vi "ConfigLCR.vi"(0 "Input parameters":T1={"Measurement type"=enum."Test", "Sensor type"=enum."HPK_8in_256", "Identifier"="test.txt", "Open after execution?"=FALSE, "Plot after execution?"=FALSE, "Display channel"=0, "Voltage Delay (s)"=0.5, "Switch Delay (s)"=0.01, "VISA resource name source"="", "VISA resource name DMM"="", "VISA resource name LCR"="", "Compliance  Level (uA)"=10.0, "Voltage Limit (V)"=1000.0, "Data storage location"="", "Scan voltages"="", "Use source as DMM?"=FALSE, "Single channel?"=FALSE, "LCR signal frequenzy (Hz)"=10.0, "DMM device"=enum."Keithley2001", "Sampling number"=1, "Use env. sensors on"=enum."Sensirion sht1x/7x"} {"Voltage Limit (V)" format="%#_13g"; "Voltage Delay (s)" format="%#_13g"; "Switch Delay (s)" format="%#_13g"}, 11 "error in (no error)":errorcluster) -> (4 "VISA resource name out":refnum<visa-resource-name>, 15 "error out":errorcluster)   [LabVIEW 2016]
uses:
  Input_parameters.ctl
  instr.lib/Agilent E4980/Agilent E4980.lvlib
panel:
  in  "Signal Frequency (1000 Hz)":dbl=10000.0
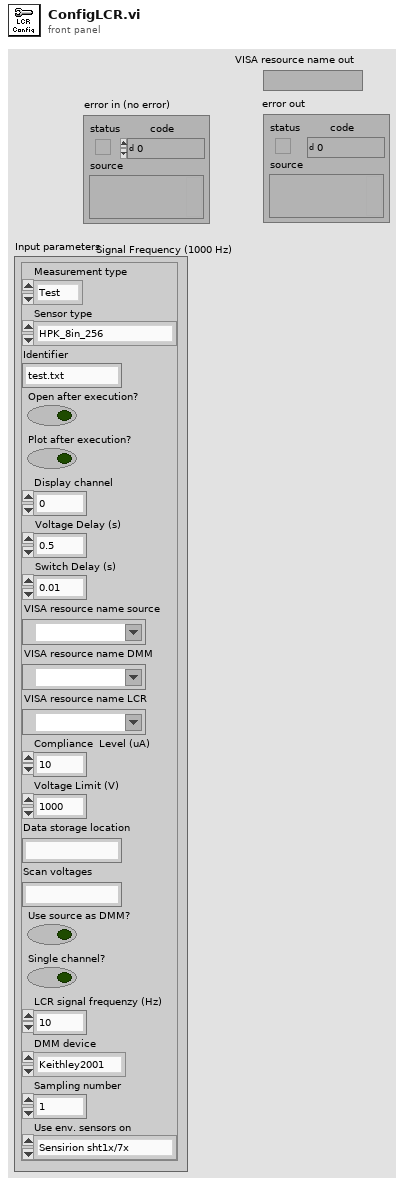
[diagram p1: front panel]
types:
  T1 = typedef "Input_parameters.ctl" = cluster{"Measurement type":enum16{"IV", "CV", "Test"}, "Sensor type":enum16{"HPK_6in_135", "HPK_8in_256", "INF_8in_256", "Diode", "HPK_6in_256"}, "Identifier":string, "Open after execution?":bool, "Plot after execution?":bool, "Display channel":i32, "Voltage Delay (s)":dbl, "Switch Delay (s)":dbl, "VISA resource name source":refnum<visa-resource-name>, "VISA resource name DMM":refnum<visa-resource-name>, "VISA resource name LCR":refnum<visa-resource-name>, "Compliance  Level (uA)":dbl, "Voltage Limit (V)":dbl, "Data storage location":string, "Scan voltages":string, "Use source as DMM?":bool, "Single channel?":bool, "LCR signal frequenzy (Hz)":dbl, "DMM device":enum16{"Keithley2001", "Keithley2450", "Keithley2410"}, "Sampling number":i32, "Use env. sensors on":enum16{"Sensirion sht1x/7x", "Switch Matrix", "Probecard"}}
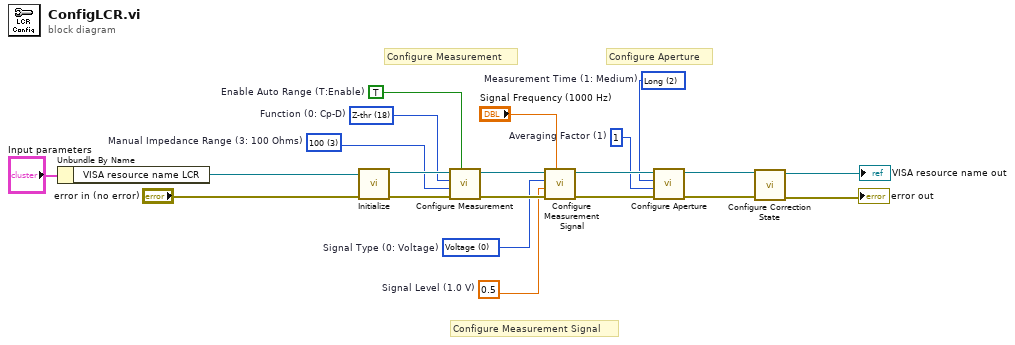
[diagram p0: block diagram]
diagram:
  w10 = u16 2 items=["Short", "Medium", "Long"]  # Measurement Time (1: Medium)
  w9 = 1  # Averaging Factor (1)
  w11 = 0.5  # Signal Level (1.0 V)
  w12 = u16 0 items=["Voltage", "Current"]  # Signal Type (0: Voltage)
  w13 = 3 items=["100m", "1", "10", "100", "300", "1K", "3K", "10K", "30K", "100K"]  # Manual Impedance Range (3: 100 Ohms)
  w14 = u16 18 items=["Cp-D", "Cp-Q", "Cp-G", "Cp-Rp", "Cs-D", "Cs-Q", "Cs-Rs", "Lp-D", "Lp-Q", "Lp-G", "Lp-Rp", "Lp-Rdc", "Ls-D", "Ls-Q", "Ls-Rs", "Ls-Rdc", "R-X", "Z-thd", "Z-thr", "G-B", "Y-thd", "Y-thr", "Vdc-Idc"]  # Function (0: Cp-D)
  w15 = TRUE  # Enable Auto Range (T:Enable)
  # "Configure Aperture"
  # "Configure Measurement Signal"
  # "Configure Measurement"
  n1 = Unbundle By Name("Input parameters") -> ("VISA resource name LCR"=w1:refnum<visa-resource-name>)
  n2 = call "Initialize.vi"("error in (no error)"="error in (no error)", "VISA resource name"=w1) -> ("error out"=w20:errorcluster, "VISA resource name out"=w21:refnum<visa-resource-name>)  [unwired: 8 in]
  n3 = call "Configure Measurement.vi"("Enable Auto Range (T:Enable)"=w15, "error in (no error)"=w20, "Manual Impedance Range (3: 100 Ohms)"=w13, "Function (0: Cp-D)"=w14, "VISA resource name"=w21) -> ("error out"=w18:errorcluster, "VISA resource name out"=w19:refnum<visa-resource-name>)  [unwired: 5 in]
  n4 = call "Configure Measurement Signal.vi"("Signal Frequency (1000 Hz)"="Signal Frequency (1000 Hz)", "error in (no error)"=w18, "Signal Level (1.0 V)"=w11, "Signal Type (0: Voltage)"=w12, "VISA resource name"=w19) -> ("error out"=w16:errorcluster, "VISA resource name out"=w17:refnum<visa-resource-name>)  [unwired: 5 in]
  n5 = call "Configure Aperture.vi"("error in (no error)"=w16, "Averaging Factor (1)"=w9, "Measurement Time (1: Medium)"=w10, "VISA resource name"=w17) -> ("error out"=w7:errorcluster, "VISA resource name out"=w5:refnum<visa-resource-name>)  [unwired: 6 in]
  n6 = call "Configure Correction State.vi"("error in (no error)"=w7, "VISA resource name"=w5) -> ("error out"=→"error out":errorcluster, "VISA resource name out"=→"VISA resource name out":refnum<visa-resource-name>)  [unwired: 8 in]
